vi "Web Cycler.vi"() -> ()   [LabVIEW 2009]
panel:
  in  "Array":string[](array[string])
  in  "SHDocVw.IWebBrowser2":refnum<k7>(container)
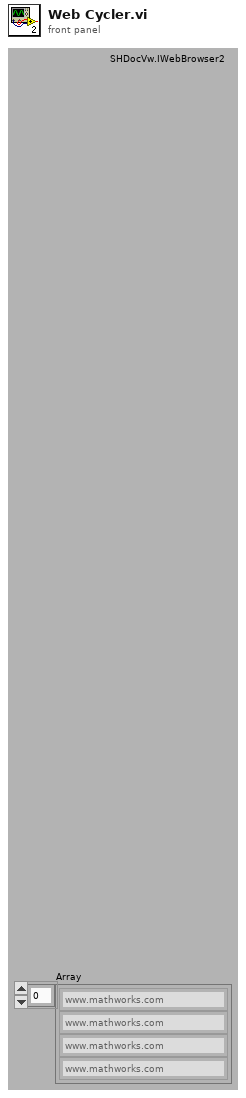
[diagram p1: front panel]
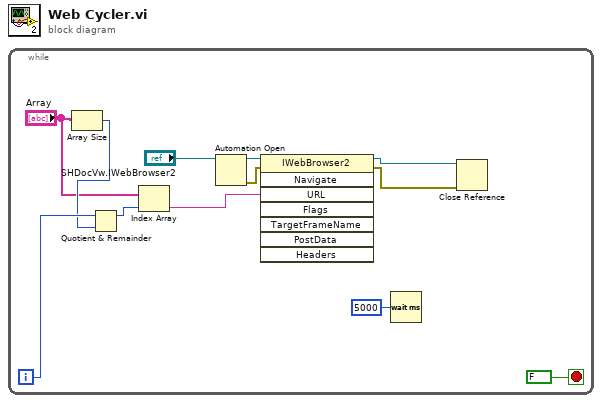
[diagram p0: block diagram]
diagram:
  n1 = while {
    i -> [w5]
    stop <- FALSE stop-if-true
    n2 = Array Size(array="Array") -> (size(s)=w4:i32)
    n3 = Quotient & Remainder(x=w5, y=w4) -> (x-y*floor(x/y)=w3:i32)  [unwired: 1 out]
    n4 = Index Array(array="Array", index=w3) -> (element=w6:string)
    n5 = Automation Open(Automation Refnum="SHDocVw.IWebBrowser2") -> (Automation Refnum=w12:refnum<k7>, error out=w11:errorcluster)  [unwired: 3 in]
    n6 = invoke class="IWebBrowser2" method="Navigate"(reference=w12, error in=w11, "URL"=w6) -> (reference out=w9:refnum<k7>, error out=w8:errorcluster)  [unwired: 5 in, 6 out]
    n7 = Wait (ms)(milliseconds to wait=u32 5000) -> ()  [unwired: 1 out]
    n8 = Close Reference(reference=w9, error in (no error)=w8) -> ()  [unwired: 1 out]
  }
